vi "Status Page.vi"(8 "Error in":errorcluster, 11 "INL DNL Test in":refnum<class "INL DNL Test.lvclass">) -> (0 "Error out":errorcluster, 3 "INL DNL Test out":refnum<class "INL DNL Test.lvclass">)   [LabVIEW 2020, in "INL DNL Test.lvclass"]
doc: "Status page which displays the DNL and INL results in graph. It also plots the transfer function and plot it in XY graph."
uses:
  INL DNL Test.lvclass
  D:/SDLC/Class/INL DNL Test/Test/Parent/Test.lvclass
  Typedef/User event controls.ctl
  Typedef/Queue Operation.ctl
  Device/Parent/Typedef/Data Cluster.ctl
  Device/Parent/Device.lvclass
  DNL INL Test.lvlib
panel:
  in  "Tab Control":enum32{"Status and graph", "Transfer Function"}(tab)
  out "INL Plot":cluster{"X Values":dbl[], "Y Values":dbl[]}(graph)
  out "DNL Plot":T1(graph)
  in  "Show Tranfer Function":bool
  out "INL":dbl
  out "DNL":dbl
  out "Code":i32
  out "Transfer Function":T2(graph)
  in  "Show DNL INL graph":bool
  # "Note:\nClick run test button to calculate and plot results in graph"
  # "Status and Graph"
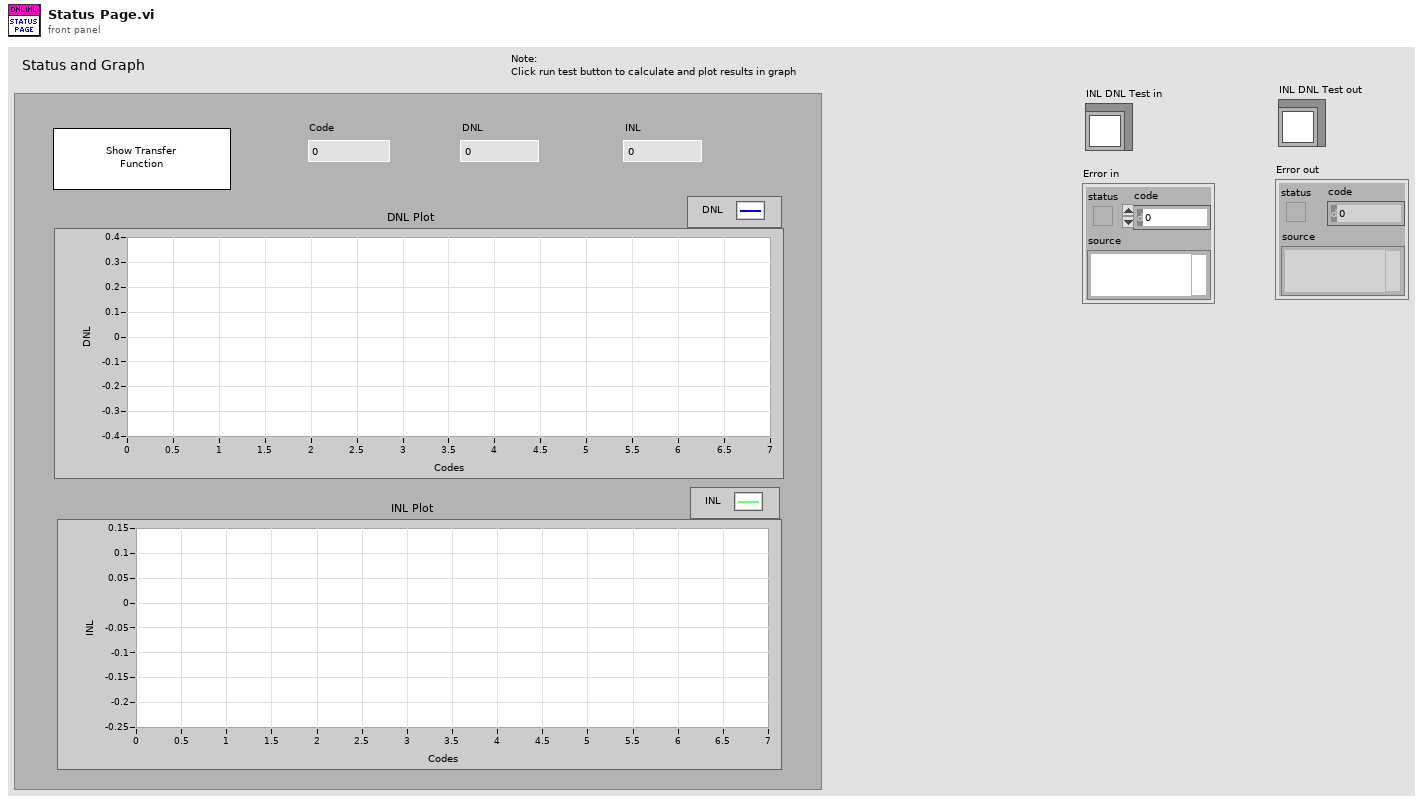
[diagram p1: front panel]
types:
  T1 = cluster{"Ideal Values":dbl[], "Deviated Values":dbl[]}
  T2 = cluster{"Ideal Vlaues":dbl[], "Deviated Values":dbl[]}[]
  T3 = typedef "DNL INL Test.lvlib/Queue Operation.ctl" = enum16{"Create Queue", "Enqueue", "Dequeue", "Enstack", "Flush Queue", "Release Queue"}
  T4 = typedef "DNL INL Test.lvlib/User event controls.ctl" = enum16{"Create", "Generate", "Run Test", "Get Ref", "Destroy"}
  T5 = typedef "Device.lvclass/Data Cluster.ctl" = cluster{"X Values":dbl[], "Y Values":dbl[]}
  T6 = enum16{"open", "replace", "create", "open or create", "replace or create", "replace or create with confirmation"}
  T7 = typedef "LVPoint32TypeDef.ctl" = cluster{"Horizontal":i32, "Vertical":i32}
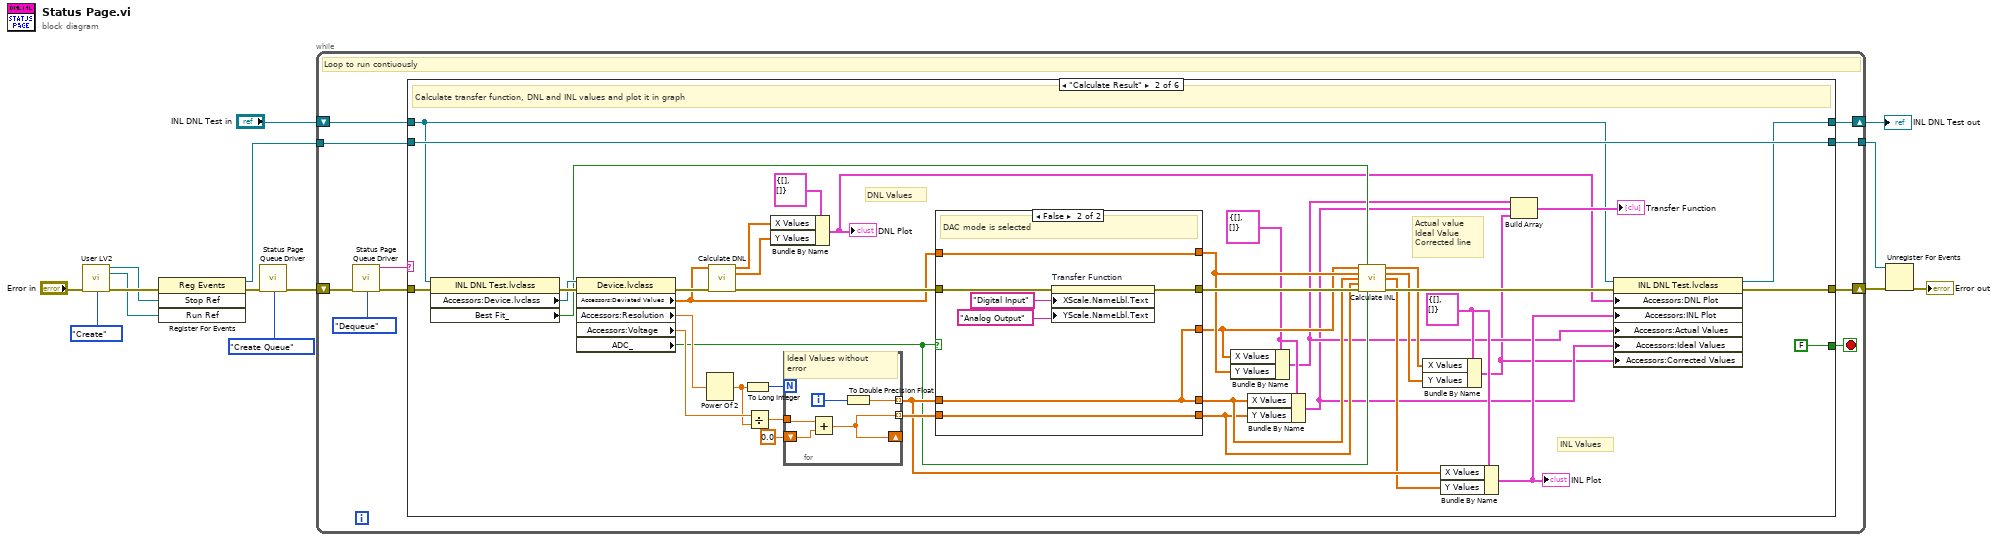
[diagram p0: block diagram]
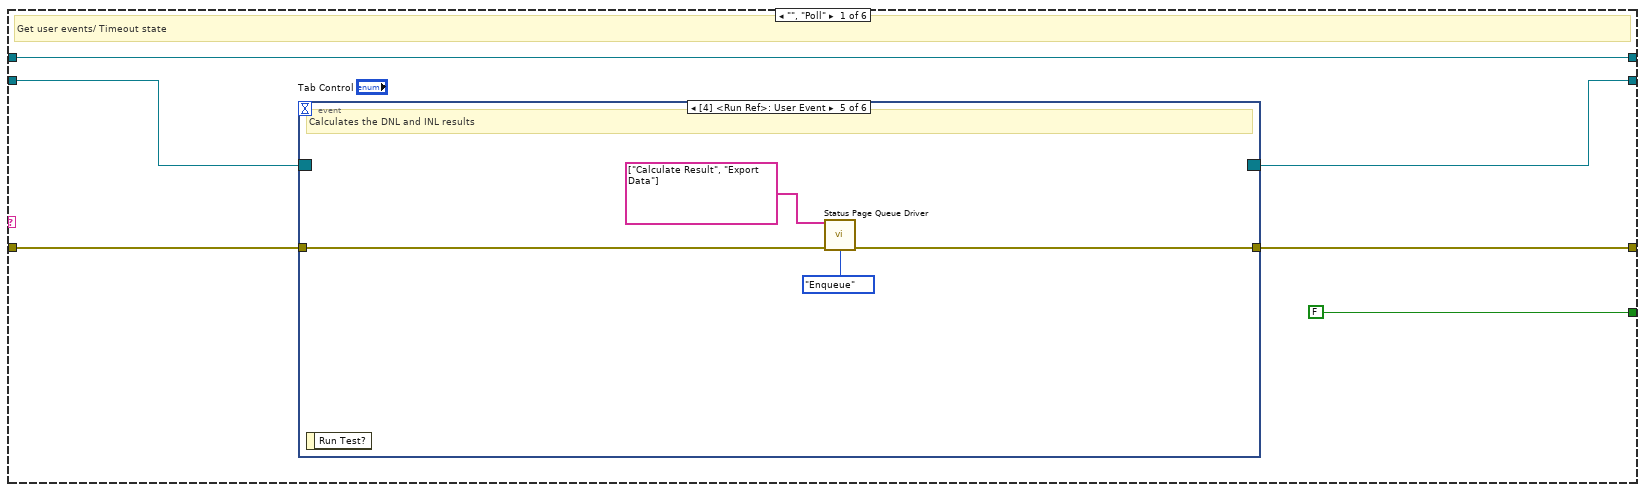
[diagram p2: hidden frame]
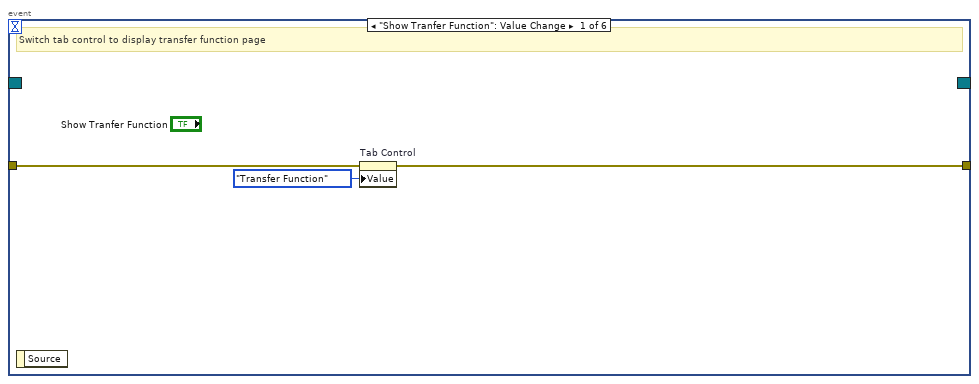
[diagram p3: hidden frame]
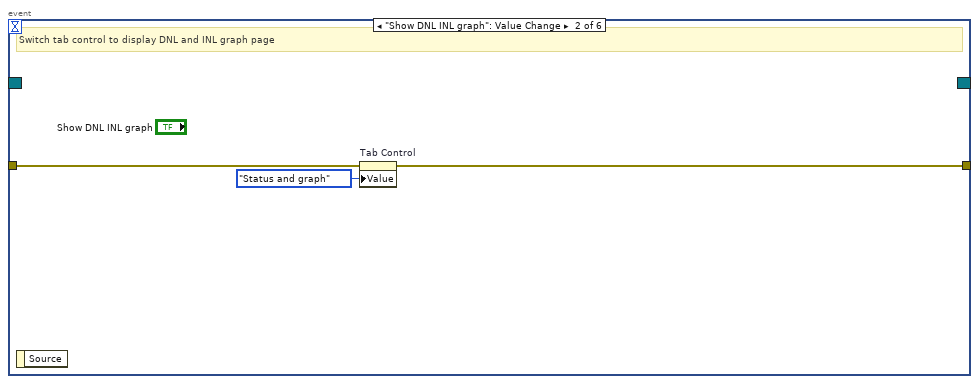
[diagram p4: hidden frame]
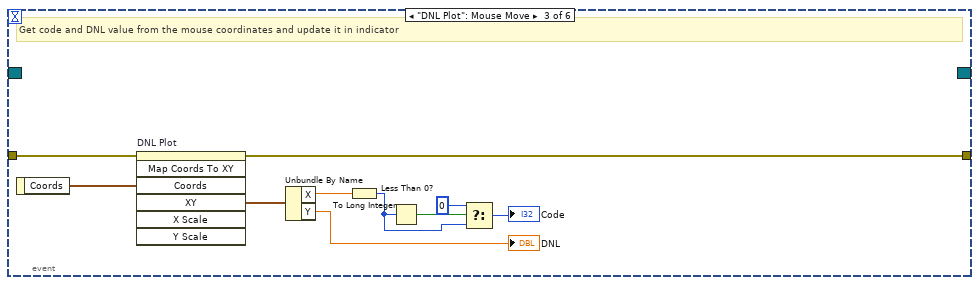
[diagram p5: hidden frame]
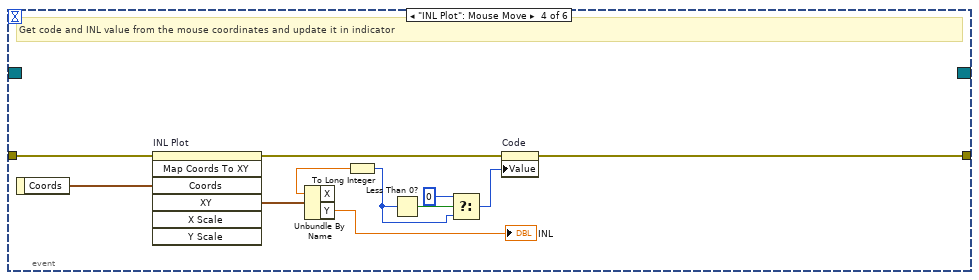
[diagram p6: hidden frame]
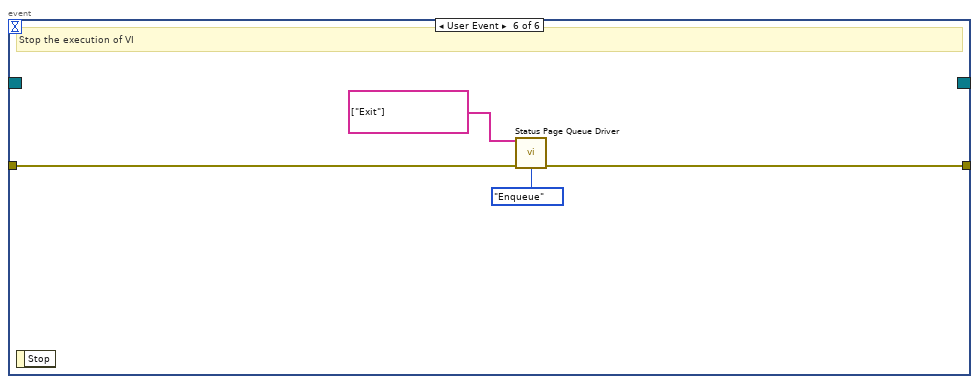
[diagram p7: hidden frame]
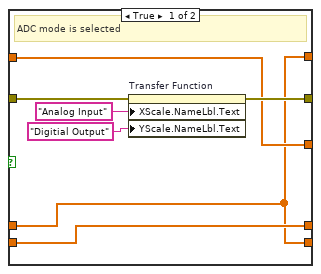
[diagram p8: hidden frame]
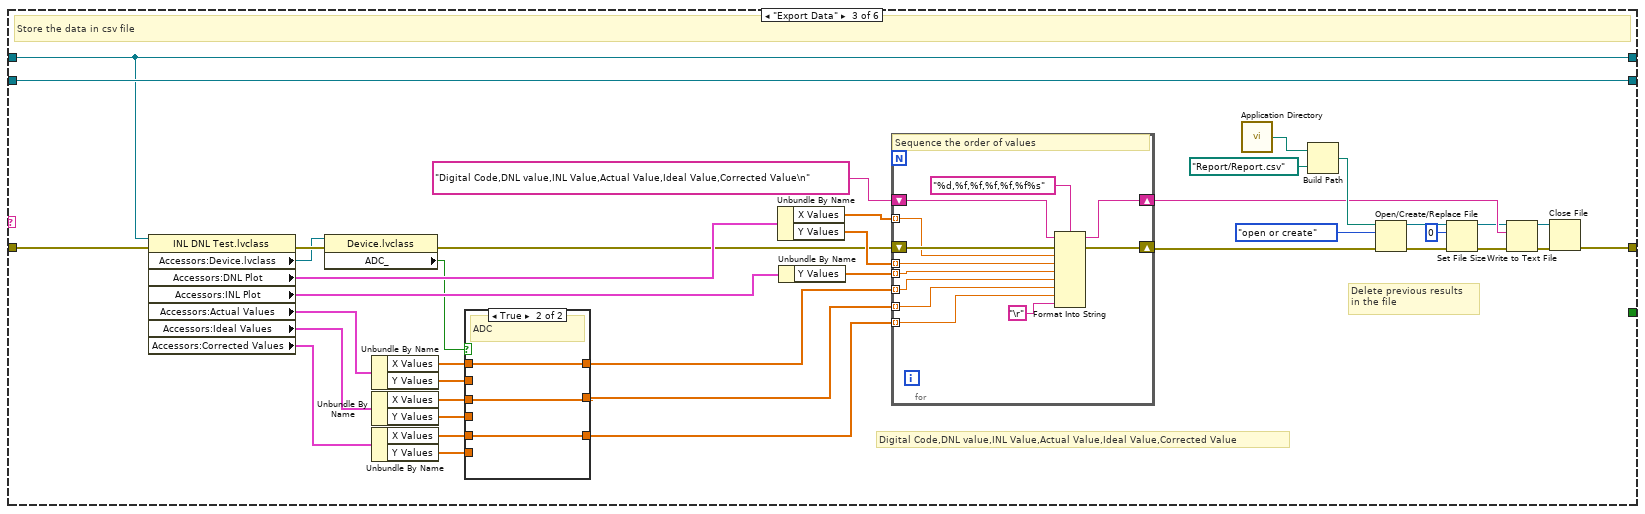
[diagram p9: hidden frame]
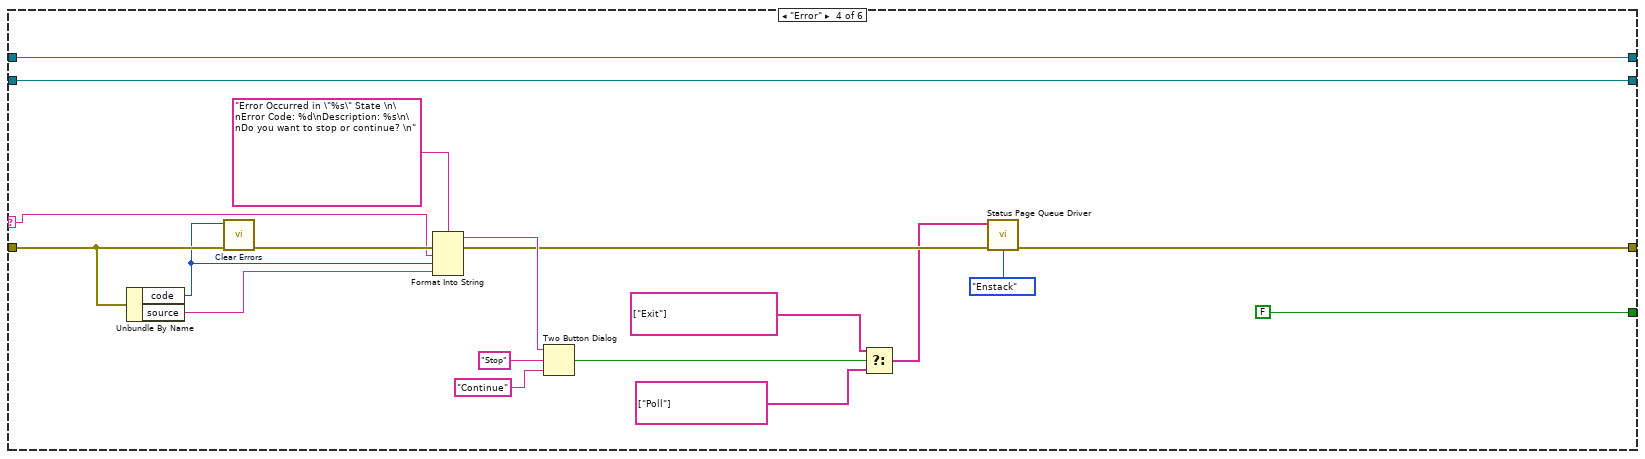
[diagram p11: hidden frame]
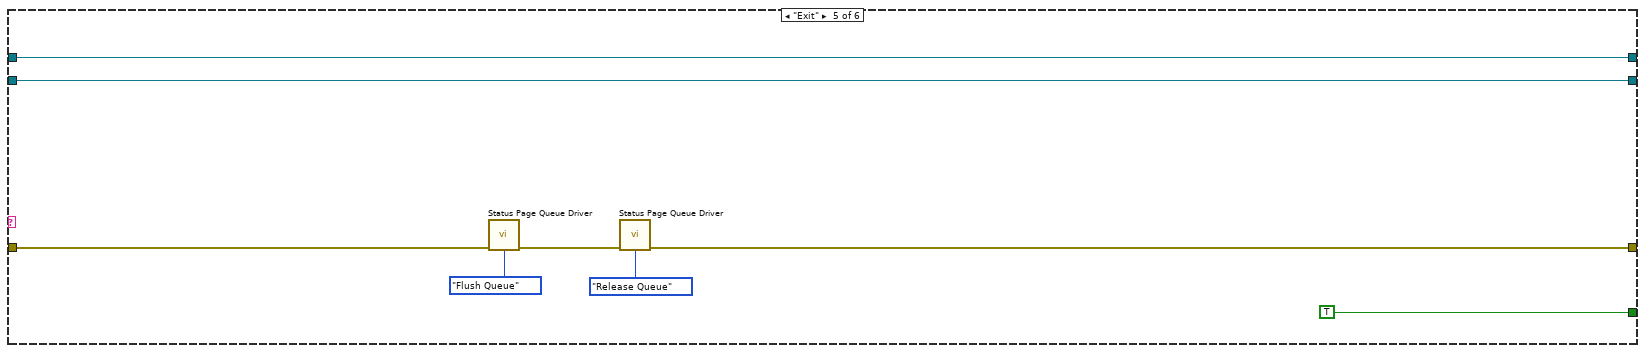
[diagram p12: hidden frame]
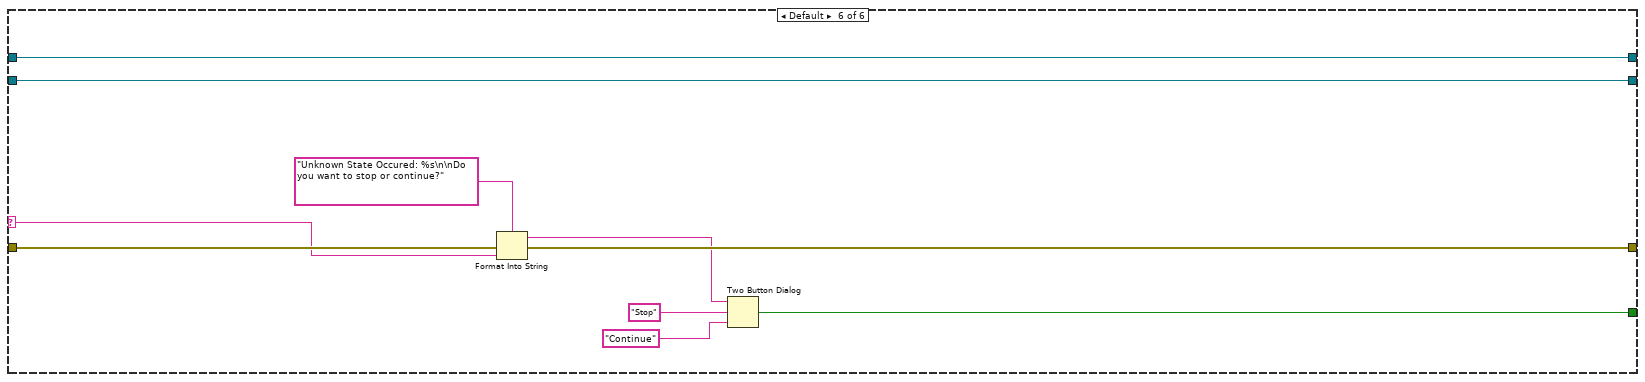
[diagram p13: hidden frame]
diagram:
  n1 = call "User LV2.vi"("Error In"="Error in", "User event controls"=User_event_controls."Create") -> ("Stop Ref"=w11:refnum<user-event>, "Run Ref"=w4:refnum<user-event>, "Error Out"=w12:errorcluster)  [unwired: 11 in]
  n2 = register-events(error in=w12, w11, w4) -> (reference out=w10:refnum<event-registration>, error out=w3:errorcluster)  [unwired: 1 in]
  n3 = call "Status Page Queue Driver.vi"("Error in"=w3, "Queue Operation"=Queue_Operation."Create Queue") -> ("Error out"=w1:errorcluster)  [unwired: 12 in, 1 out]
  n4 = while {
    shift-right: [w24] -> w9
    shift-left: w1 -> [w16]
    tunnel: w10 -> [w23]
    tunnel: [w21] -> w7
    shift-right: [w19] -> w5
    shift-left: "INL DNL Test in" -> [w20]
    stop <- w22 stop-if-true
    # "Loop to run contiuously"
    n5 = call "Status Page Queue Driver.vi"("Error in"=w16, "Queue Operation"=Queue_Operation."Dequeue") -> ("Dequeue Element"=w15:string, "Error out"=w17:errorcluster)  [unwired: 12 in]
    n6 = case shown="\"Calculate Result\"" w15 {
      selector: w15 -> [_ _ _ w196 _ w214]
      tunnel: w17 -> [w30 w99 w164 w198 w207 w219]
      tunnel: [w29 w73 w158 w188 w203 w216] -> w24
      tunnel: w23 -> [w28 w97 w163 w201 w209 w218]
      tunnel: [FALSE ("Stop") FALSE ("Stop") _ FALSE ("T button?") TRUE ("Stop") w210] -> w22
      tunnel: [w27 w97 w163 w201 w209 w218] -> w21
      tunnel: w20 -> [w25 w72 w162 w200 w208 w217]
      tunnel: [w25 w70 w162 w200 w208 w217] -> w19
      frame "", "Poll" {
        # "Get user events/ Timeout state"
        n7 = event shown="[4] <Run Ref>: User Event" {
          selector: w28 -> [_ _ _ _ _ _]
          dyn-events: [_ _ _ _ _ _] -> w27
          timeout: _ -> [_ _ _ _ _ _]
          tunnel: w30 -> [w33 w36 w46 w57 w61 w65]
          tunnel: [w32 w35 w45 w52 w60 w64] -> w29
          event "Show Tranfer Function": Value Change {
            # "Switch tab control to display transfer function page"
            n8 = event-data() -> ()  [unwired: 1 in, 1 out]
            n9 = property on="Tab Control" class="TabCtl (strict)"(error in=w33, "Value"=enum32{"Status and graph", "Transfer Function"}."Transfer Function" ("Tab Control")) -> (error out=w32:errorcluster)  [unwired: 1 in, 1 out]
          }
          event "Show DNL INL graph": Value Change {
            # "Switch tab control to display DNL and INL graph page"
            n10 = event-data() -> ()  [unwired: 1 in, 1 out]
            n11 = property on="Tab Control" class="TabCtl (strict)"(error in=w36, "Value"=enum32{"Status and graph", "Transfer Function"}."Status and graph" ("Tab Control")) -> (error out=w35:errorcluster)  [unwired: 1 in, 1 out]
          }
          event "DNL Plot": Mouse Move {
            # "Get code and DNL value from the mouse coordinates and update it in indicator"
            n12 = event-data() -> ("Coords"=w44:T7)  [unwired: 1 in]
            n13 = invoke on="DNL Plot" class="XYGraph (strict)" method="Map Coords To XY"(error in=w46, "Coords"=w44) -> (error out=w45:errorcluster, "XY"=w43:cluster{"X":dbl, "Y":dbl})  [unwired: 5 in, 5 out]
            n14 = Unbundle By Name(w43) -> ("X"=w42:dbl, "Y"=→"DNL":dbl)
            n15 = To Long Integer(number=w42) -> (32bit integer=w39:i32)
            n16 = Less Than 0?(x=w39) -> (x < 0?=w40:bool)
            n17 = Select(t=0, s=w40, f=w39) -> (s? t:f=→"Code":i32)
          }
          event "INL Plot": Mouse Move {
            # "Get code and INL value from the mouse coordinates and update it in indicator"
            n18 = event-data() -> ("Coords"=w55:T7)  [unwired: 1 in]
            n19 = invoke on="INL Plot" class="XYGraph (strict)" method="Map Coords To XY"(error in=w57, "Coords"=w55) -> (error out=w56:errorcluster, "XY"=w54:cluster{"X":dbl, "Y":dbl})  [unwired: 5 in, 5 out]
            n20 = Unbundle By Name(w54) -> ("X"=w51:dbl, "Y"=→"INL":dbl)
            n21 = To Long Integer(number=w51) -> (32bit integer=w49:i32)
            n22 = Less Than 0?(x=w49) -> (x < 0?=w50:bool)
            n23 = Select(t=0, s=w50, f=w49) -> (s? t:f=w47:i32)
            n24 = property on="Code" class="DigNum (strict)"(error in=w56, "Value"=w47) -> (error out=w52:errorcluster)  [unwired: 1 in, 1 out]
          }
          event User Event {
            # "Calculates the DNL and INL results"
            n25 = event-data() -> ()  [unwired: 1 in, 1 out]
            n26 = call "Status Page Queue Driver.vi"("States"=string[] ["Calculate Result", "Export Data"], "Error in"=w61, "Queue Operation"=Queue_Operation."Enqueue") -> ("Error out"=w60:errorcluster)  [unwired: 11 in, 1 out]
          }
          event User Event {
            # "Stop the execution of VI"
            n27 = event-data() -> ()  [unwired: 1 in, 1 out]
            n28 = call "Status Page Queue Driver.vi"("States"=string[] ["Exit"], "Error in"=w65, "Queue Operation"=Queue_Operation."Enqueue") -> ("Error out"=w64:errorcluster)  [unwired: 11 in, 1 out]
          }
        }
      }
      frame "Calculate Result" {
        w76 = T5 {"X Values"=[], "Y Values"=[]} ("Cluster")
        w95 = T5 {"X Values"=[], "Y Values"=[]} ("Cluster")
        # "INL Values"
        # "Actual value\nIdeal Value\nCorrected line"
        # "DNL Values"
        # "Calculate transfer function, DNL and INL values and plot it in graph"
        n29 = property class="INL DNL Test.lvclass"(reference=w72, error in=w99) -> (error out=w106:errorcluster, "Accessors:Device.lvclass"=w105:refnum<class "Device.lvclass">, "Best Fit_"=w80:bool)  [unwired: 1 out]
        n30 = property class="Device.lvclass"(reference=w105, error in=w106) -> (error out=w92:errorcluster, "Accessors:Deviated Values"=w87:dbl[], "Accessors:Resolution"=w104:dbl, "Accessors:Voltage"=w102:dbl, "ADC_"=w79:bool)  [unwired: 1 out]
        n31 = Power Of 2(x=w104) -> (2^x=w88:dbl)
        n32 = call "Calculate DNL.vi"("Deviated Values"=w87, "Error in"=w92) -> ("Codes"=w90:dbl[], "DNL Values"=w89:dbl[], "Error out"=w91:errorcluster)  [unwired: 11 in]
        n33 = To Long Integer(number=w88) -> (32bit integer=w103:i32)
        n34 = Divide(x=w102, y=w88) -> (x/y=w101:dbl)
        n35 = Bundle By Name(cluster=T5 {"X Values"=[], "Y Values"=[]} ("Cluster"), "X Values"=w90, "Y Values"=w89) -> (w71:T5)
        "DNL Plot" <- w71
        n36 = for {
          N: w103 -> [_]
          tunnel: w101 -> [w111]
          shift-right: [w109] -> _
          shift-left: 0.0 ("y") -> [w110]
          tunnel: [w109] -> w93 mode=indexing
          tunnel: [w107] -> w86 mode=indexing
          i -> [w108]
          # "Ideal Values without error"
          n37 = Add(x=w111, y=w110) -> (x+y=w109:dbl)
          n38 = To Double Precision Float(number=w108) -> (double precision float=w107:dbl)
        }
        n39 = case shown="False" w79 {
          tunnel: w91 -> [w118 w125]
          tunnel: w86 -> [w112 w121]
          tunnel: w93 -> [w114 w119]
          tunnel: [w117 w124] -> w85
          tunnel: [w114 w121] -> w82
          tunnel: [w112 w119] -> w81
          tunnel: w87 -> [w113 w120]
          tunnel: [w112 w120] -> w83
          tunnel: [w113 w121] -> w78
          frame True {
            # "ADC mode is selected"
            n40 = property on="Transfer Function" class="XYGraph (strict)"(error in=w118, "XScale.NameLbl.Text"="Analog Input" ("X Scale.Name Label.Text"), "YScale.NameLbl.Text"="Digitial Output" ("Y Scale.Name Label.Text")) -> (error out=w117:errorcluster)  [unwired: 1 in, 1 out]
          }
          frame False {
            # "DAC mode is selected"
            n41 = property on="Transfer Function" class="XYGraph (strict)"(error in=w125, "XScale.NameLbl.Text"="Digital Input" ("X Scale.Name Label.Text"), "YScale.NameLbl.Text"="Analog Output" ("Y Scale.Name Label.Text")) -> (error out=w124:errorcluster)  [unwired: 1 in, 1 out]
          }
        }
        n42 = Bundle By Name(cluster=w76, "X Values"=w78, "Y Values"=w83) -> (w68:T5)
        n43 = Bundle By Name(cluster=w76, "X Values"=w82, "Y Values"=w81) -> (w67:T5)
        n44 = call "Calculate INL.vi"("Actual X"=w78, "Best Fit?"=w80, "Actual Y"=w83, "Ideal X"=w82, "Ideal Y"=w81, "Error in"=w85, "ADC?"=w79) -> ("INL X Plot values"=w75:dbl[], "INL Y Plot Values"=w74:dbl[], "INL Result values"=w77:dbl[], "Error out"=w84:errorcluster)  [unwired: 5 in]
        n45 = Bundle By Name(cluster=w95, "X Values"=w75, "Y Values"=w74) -> (w66:T5)
        n46 = Bundle By Name(cluster=w95, "X Values"=w86, "Y Values"=w77) -> (w69:T5)
        "INL Plot" <- w69
        n47 = Build Array(w68, w67, w66) -> (→"Transfer Function":T5[])
        n48 = property class="INL DNL Test.lvclass"(reference=w72, error in=w84, "Accessors:DNL Plot"=w71, "Accessors:INL Plot"=w69, "Accessors:Actual Values"=w68, "Accessors:Ideal Values "=w67, "Accessors:Corrected Values"=w66) -> (reference out=w70:refnum<class "INL DNL Test.lvclass">, error out=w73:errorcluster)
      }
      frame "Export Data" {
        # "Delete previous results\nin the file"
        # "Digital Code,DNL value,INL Value,Actual Value,Ideal Value,Corrected Value"
        # "Store the data in csv file"
        n49 = property class="INL DNL Test.lvclass"(reference=w162, error in=w164) -> (error out=w159:errorcluster, "Accessors:Device.lvclass"=w148:refnum<class "Device.lvclass">, "Accessors:DNL Plot"=w150:T5, "Accessors:INL Plot"=w153:T5, "Accessors:Actual Values"=w146:T5, "Accessors:Ideal Values "=w143:T5, "Accessors:Corrected Values"=w136:T5)  [unwired: 1 out]
        n50 = property class="Device.lvclass"(reference=w148, error in=w159) -> (error out=w149:errorcluster, "ADC_"=w147:bool)  [unwired: 1 out]
        n51 = Unbundle By Name(w146) -> ("X Values"=w145:dbl[], "Y Values"=w144:dbl[])
        n52 = Unbundle By Name(w143) -> ("X Values"=w142:dbl[], "Y Values"=w141:dbl[])
        n53 = Unbundle By Name(w136) -> ("X Values"=w135:dbl[], "Y Values"=w134:dbl[])
        n54 = case shown="True" w147 {
          tunnel: w145 -> [_ w170]
          tunnel: w144 -> [w167 _]
          tunnel: [w167 w170] -> w140
          tunnel: w142 -> [_ w169]
          tunnel: [w166 w169] -> w139
          tunnel: w141 -> [w166 _]
          tunnel: [w165 w168] -> w133
          tunnel: w135 -> [_ w168]
          tunnel: w134 -> [w165 _]
          frame False {
            # "DAC"
          }
          frame True {
            # "ADC"
          }
        }
        n55 = Unbundle By Name(w150) -> ("X Values"=w157:dbl[], "Y Values"=w151:dbl[])
        n56 = Unbundle By Name(w153) -> ("Y Values"=w152:dbl[])
        n57 = for {
          shift-right: [w178] -> w137
          shift-left: w149 -> [w182]
          tunnel: w157 -> [w180] mode=indexing
          tunnel: w151 -> [w179] mode=indexing
          shift-right: [w177] -> w138
          shift-left: "Digital Code,DNL value,INL Value,Actual Value,Ideal Value,Corrected Value\n" -> [w176]
          tunnel: w152 -> [w175] mode=indexing
          tunnel: w140 -> [w174] mode=indexing
          tunnel: w139 -> [w173] mode=indexing
          tunnel: w133 -> [w172] mode=indexing
          # "Sequence the order of values"
          n58 = Format Into String(format string="%d,%f,%f,%f,%f,%f%s", initial string=w176, error in=w182, w180, w179, w175, w174, w173, w172, "\r") -> (resulting string=w177:string, error out=w178:errorcluster)
        }
        n59 = call <vilib>:"Application Directory.vi"() -> ("Application Directory"=w161:path)
        n60 = Build Path(base path=w161, name or relative path=path "Report/Report.csv") -> (appended path=w156:path)
        n61 = Open/Create/Replace File(file path (use dialog)=w156, error in=w137, operation (0:open)=T6."open or create") -> (refnum out=w129:refnum<file>, error out=w131:errorcluster)  [unwired: 3 in, 1 out]
        n62 = Set File Size(4:w131, 6:i64 0 ("size (in bytes)"), 7:w129) -> (0:w130:errorcluster, 3:w128:refnum<file>)
        n63 = Write to Text File(file (use dialog)=w128, text=w138, error in=w130) -> (refnum out=w154:refnum<file>, error out=w155:errorcluster)  [unwired: 1 in, 1 out]
        n64 = Close File(refnum=w154, error in=w155) -> (error out=w158:errorcluster)  [unwired: 1 out]
      }
      frame "Error" {
        n65 = Unbundle By Name(w198) -> ("code"=w195:i32, "source"=w194:string)
        n66 = call <vilib>:"Clear Errors.vi"("error in (no error)"=w198, "specific error code to clear (0: all)"=w195) -> ("error out"=w197:errorcluster)  [unwired: 4 in, 1 out]
        n67 = Format Into String(format string="Error Occurred in \"%s\" State \n\nError Code: %d\nDescription: %s\n\nDo you want to stop or continue? \n", error in=w197, w196, w195, w194) -> (resulting string=w193:string, error out=w189:errorcluster)  [unwired: 1 in]
        n68 = Two Button Dialog(message=w193, 1:"Continue" ("F button name (\"Cancel\")"), 2:"Stop" ("T button name (\"OK\")")) -> (T button?=w190:bool)
        n69 = Select(t=string[] ["Exit"] ("States"), s=w190, f=string[] ["Poll"]) -> (s? t:f=w185:string[])
        n70 = call "Status Page Queue Driver.vi"("States"=w185, "Error in"=w189, "Queue Operation"=Queue_Operation."Enstack") -> ("Error out"=w188:errorcluster)  [unwired: 11 in, 1 out]
      }
      frame "Exit" {
        n71 = call "Status Page Queue Driver.vi"("Error in"=w207, "Queue Operation"=Queue_Operation."Flush Queue") -> ("Error out"=w205:errorcluster)  [unwired: 12 in, 1 out]
        n72 = call "Status Page Queue Driver.vi"("Error in"=w205, "Queue Operation"=Queue_Operation."Release Queue") -> ("Error out"=w203:errorcluster)  [unwired: 12 in, 1 out]
      }
      frame Default {
        n73 = Format Into String(format string="Unknown State Occured: %s\n\nDo you want to stop or continue?", error in=w219, w214) -> (resulting string=w213:string, error out=w216:errorcluster)  [unwired: 1 in]
        n74 = Two Button Dialog(message=w213, 1:"Continue" ("F button name (\"Cancel\")"), 2:"Stop" ("T button name (\"OK\")")) -> (T button?=w210:bool)
      }
    }
  }
  "INL DNL Test out" <- w5
  n75 = Unregister For Events(event registration refnum=w7, error in=w9) -> (error out=→"Error out":errorcluster)
